vi "getGlyphFile.vi"(8 "error in (no error)":errorcluster, 11 "Channel in":refnum<class "Channel.lvclass">) -> (0 "error out":errorcluster, 2 "Glyph File":string, 3 "Channel out":refnum<class "Channel.lvclass">)   [LabVIEW 2013, in "Channel.lvclass"]
doc: "Dynamic Dispatch VI. Returns the name of the glyph file to be used as a glyph in the tree control. A empty string means no glyph."
uses:
  Channel.lvclass
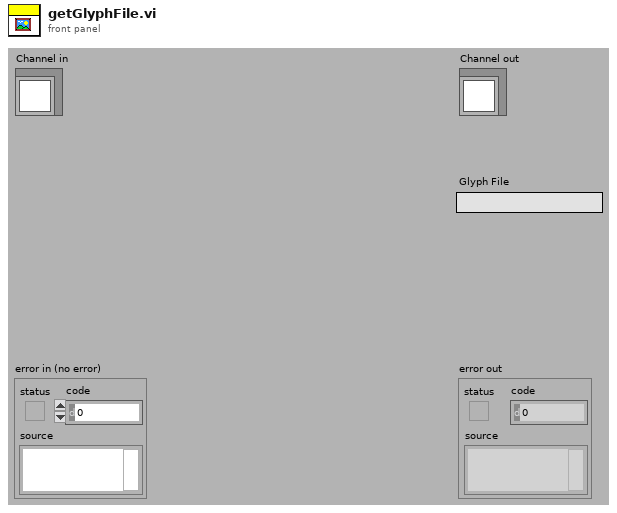
[diagram p1: front panel]
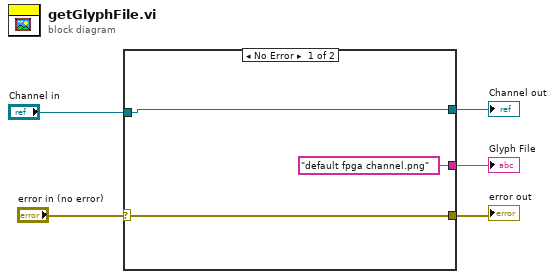
[diagram p0: block diagram]
diagram:
  n1 = case shown="No Error" "error in (no error)" {
    selector: "error in (no error)" -> [w7 w9]
    tunnel: "Channel in" -> [w8 w10]
    tunnel: [w8 w10] -> w3
    tunnel: [w7 w9] -> w2
    tunnel: ["default fpga channel.png" _] -> w1
    frame No Error {
    }
    frame Error {
    }
  }
  "error out" <- w2
  "Channel out" <- w3
  "Glyph File" <- w1
